vi "FlpLib Integrator 4.vi"(1 "dt":sgl, 7 "dx":sgl, 12 "initial":sgl format="%#_13g") -> (8 "x":sgl)   [LabVIEW 2017]
uses:
  <userlib>/_NI FLP Library/FPGA/outsideSCTL/FlpLib Multiply Shared Instance 4.vi
  <userlib>/_NI FLP Library/FPGA/outsideSCTL/FlpLib Add Shared Instance 4.vi
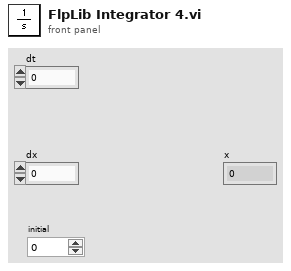
[diagram p1: front panel]
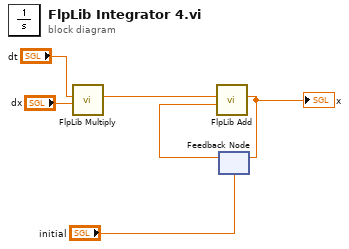
[diagram p0: block diagram]
diagram:
  n1 = call-poly <userlib>:"FlpLib Multiply.vi"("y"="dx", "x"="dt") -> ("x*y"=w4:sgl)  [unwired: 5 in]
  n2 = feedback #1("initial") -> (w3:sgl)
  n3 = call-poly <userlib>:"FlpLib Add.vi"("y"=w3, "x"=w4) -> ("x+y"=w2:sgl)  [unwired: 5 in]
  "x" <- w2
  n4 = feedback-in #1(w2) -> ()
